vi "Create Resources.vi"() -> (2 "Oscillator Address Space out":refnum<class "Oscillator.lvclass">, 3 "Subsystem out":refnum<class "Single Address Space Collection.lvclass">)   [LabVIEW 2017, in "Oscillator.lvlib" / "Oscillator.lvclass"]
uses:
  Oscillator.lvclass
  C:/Program Files (x86)/National Instruments/LabVIEW 2017/instr.lib/_niInstr/Instruction Framework/v1/FPGA/Interfaces/Address Space/Address Space.lvclass
  <instrlib>/_niInstr/Instruction Framework/v1/FPGA/Helper Classes/Single Address Space Collection/Single Address Space Collection.lvclass
  <instrlib>/_niInstr/Instruction Framework/v1/FPGA/Interfaces/Address Space/Address Space.lvclass
  Oscillator.lvclass/Oscillator.ctl
  <vilib>/rvi/DataTransferAndStorage/Container/Common/niFpgaContainerGetUniqueNameForEmu.vi
  <vilib>/rvi/DataTransferAndStorage/Container/Common/niFpgaContainerSetEmuInfo.vi
  <vilib>/rvi/eio/common/nirviEmuReportErrorAndStop.vi
  <vilib>/rvi/LocalResourceManager/LocalResourceManager.xnode
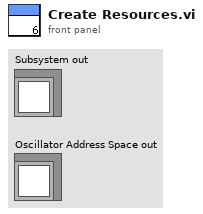
[diagram p1: front panel]
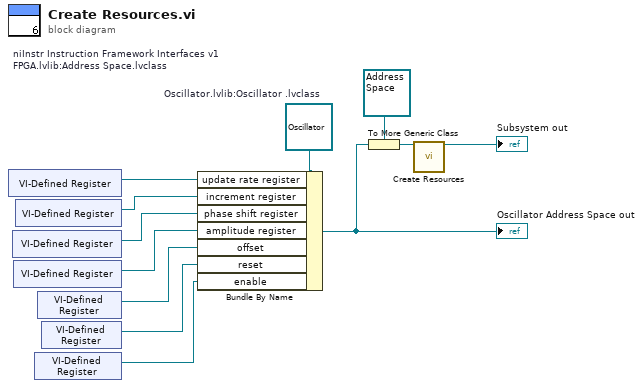
[diagram p0: block diagram]
diagram:
  w6 = refnum<class "Address Space.lvclass"> refnum  # niInstr Instruction Framework Interfaces v1 FPGA.lvlib:Address Space.lvclass
  w12 = refnum<class "Oscillator.lvclass"> refnum  # Oscillator.lvlib:Oscillator .lvclass
  n1 = xnode "VI-Defined Register"() -> ("Register Out"=w4:refnum<k21>)
  n2 = xnode "VI-Defined Register"() -> ("Register Out"=w10:refnum<k21>)
  n3 = xnode "VI-Defined Register"() -> ("Register Out"=w9:refnum<k21>)
  n4 = xnode "VI-Defined Register"() -> ("Register Out"=w11:refnum<k21>)
  n5 = xnode "VI-Defined Register"() -> ("Register Out"=w1:refnum<k21>)
  n6 = xnode "VI-Defined Register"() -> ("Register Out"=w3:refnum<k21>)
  n7 = xnode "VI-Defined Register"() -> ("Register Out"=w2:refnum<k21>)
  n8 = Bundle By Name(cluster=w12, "update rate register"=w4, "increment register"=w11, "phase shift register"=w10, "amplitude register"=w9, "offset"=w3, "reset"=w2, "enable"=w1) -> (w7:refnum<class "Oscillator.lvclass">)
  "Oscillator Address Space out" <- w7
  n9 = To More Generic Class(target class=w6, reference=w7) -> (generic class reference=w8:refnum<class "Address Space.lvclass">)
  n10 = call <instrlib>:"Create Resources.vi"("address space"=w8) -> ("single address space collection"=→"Subsystem out":refnum<class "Single Address Space Collection.lvclass">)  [unwired: 14 in]
